vi "CRYSet Run Project Front Panel.vi"(11 "Vi Ref in":refnum<vi> caption="Vi Ref") -> (3 "Vi Ref out":refnum<vi> caption="Vi Ref")   [LabVIEW 2013]
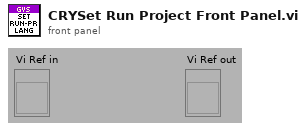
[diagram p1: front panel]
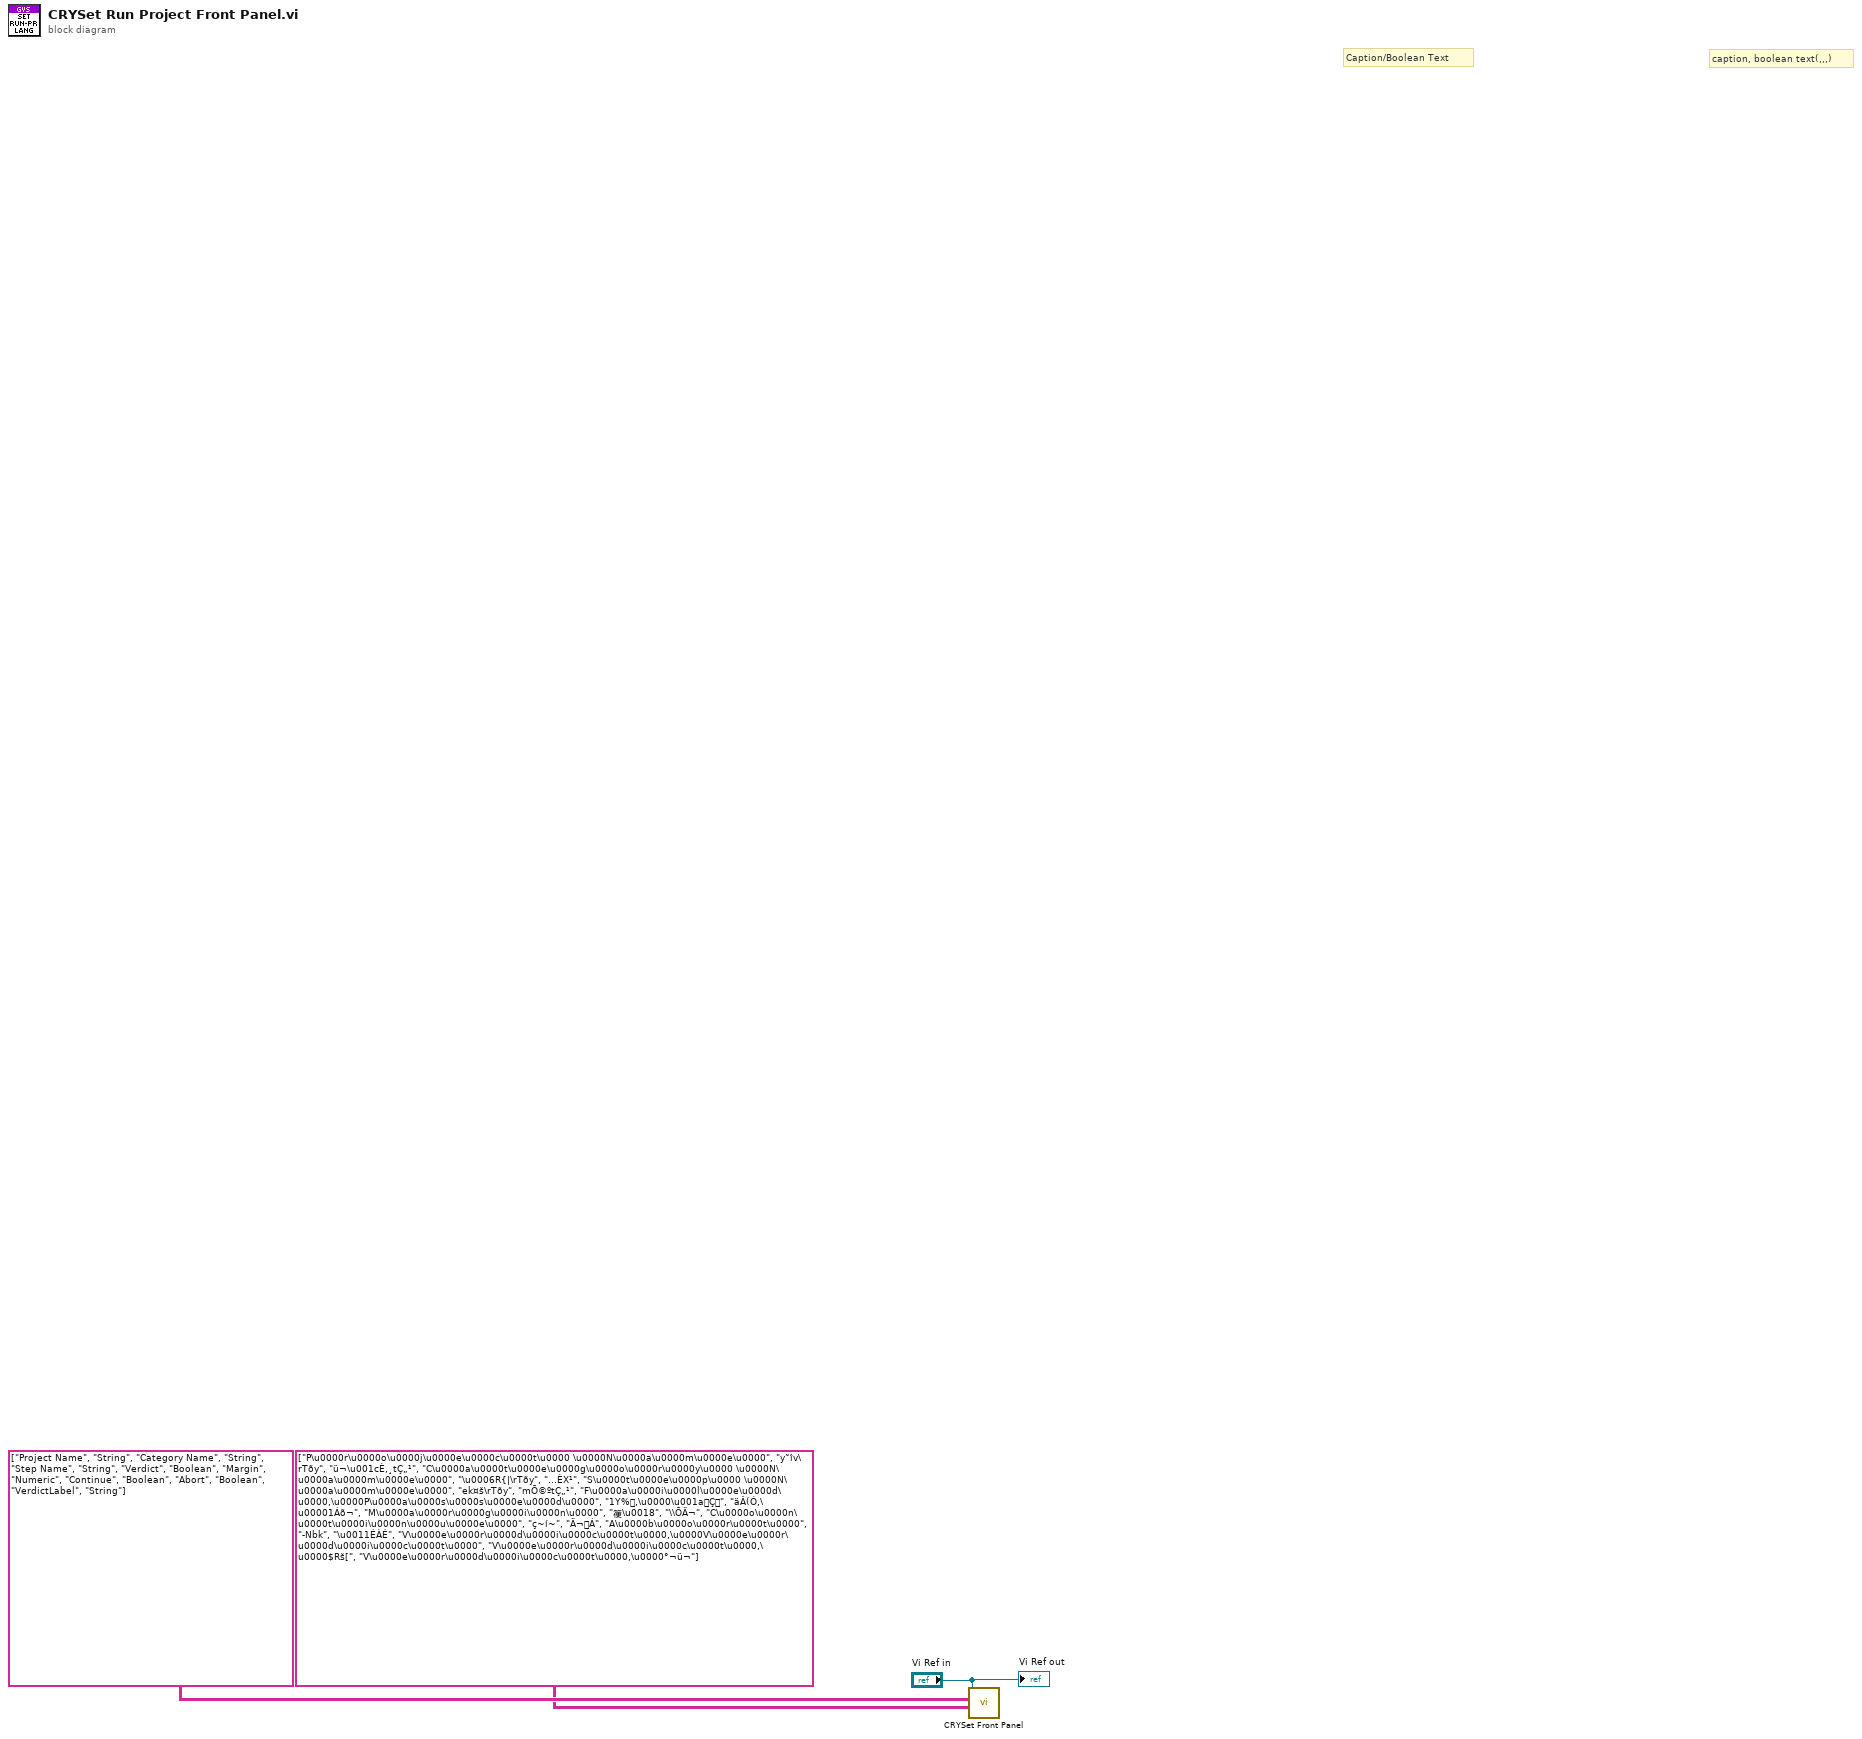
[diagram p0: block diagram]
diagram:
  # "caption, boolean text(,,,)"
  # "Caption/Boolean Text"
  n1 = call "CRYSet Front Panel.vi"("Caption(Boolean Text)"=string[][] [["P\u0000r\u0000o\u0000j\u0000e\u0000c\u0000t\u0000 \u0000N\u0000a\u0000m\u0000e\u0000", "y˜îv\rTðy", "ü¬\u001cÈ,¸tÇ„¹"], ["C\u0000a\u0000t\u0000e\u0000g\u0000o\u0000r\u0000y\u0000 \u0000N\u0000a\u0000m\u0000e\u0000", "\u0006R{|\rTðy", "…ÈX¹"], ["S\u0000t\u0000e\u0000p\u0000 \u0000N\u0000a\u0000m\u0000e\u0000", "ek¤š\rTðy", "mÕ©ºtÇ„¹"], ["F\u0000a\u0000i\u0000l\u0000e\u0000d\u0000,\u0000P\u0000a\u0000s\u0000s\u0000e\u0000d\u0000", "1Y%,\u0000\u001aÇ", "äÂ(Ó,\u00001Áõ¬"], ["M\u0000a\u0000r\u0000g\u0000i\u0000n\u0000", "箯\u0018", "\\ÕÄ¬"], ["C\u0000o\u0000n\u0000t\u0000i\u0000n\u0000u\u0000e\u0000", "ç~í~", "Ä¬Á"], ["A\u0000b\u0000o\u0000r\u0000t\u0000", "-Nbk", "\u0011ÉÀÉ"], ["V\u0000e\u0000r\u0000d\u0000i\u0000c\u0000t\u0000,\u0000V\u0000e\u0000r\u0000d\u0000i\u0000c\u0000t\u0000", "V\u0000e\u0000r\u0000d\u0000i\u0000c\u0000t\u0000,\u0000$Rš[", "V\u0000e\u0000r\u0000d\u0000i\u0000c\u0000t\u0000,\u0000°¬ü¬"]], "Control ID and Type(Label Name, Type)"=string[][] [["Project Name", "String"], ["Category Name", "String"], ["Step Name", "String"], ["Verdict", "Boolean"], ["Margin", "Numeric"], ["Continue", "Boolean"], ["Abort", "Boolean"], ["VerdictLabel", "String"]], "Vi Ref"="Vi Ref in") -> ()  [unwired: 9 in]
  "Vi Ref out" <- "Vi Ref in"
